vi "Main Interface.vi"() -> ()   [LabVIEW 2015]
uses:
  Ctrls/Data operation control.ctl
  <vilib>/Utility/error.llb/DialogType.ctl
  <vilib>/DAQmx/read.llb/DAQmx Read (Counter U32 1Chan 1Samp).vi
  <vilib>/DAQmx/create/channels.llb/DAQmx Create Channel (CI-Count Edges).vi
  <vilib>/DAQmx/miscellaneous.llb/DAQmx Fill In Error Info.vi
  <vilib>/Waveform/WDTFileIO.llb/Export Waveform To Spreadsheet File.vi
  <resource>/objmgr/daqmx.rc
panel:
  in  "Threshold value (mV)":i16=150
  in  "Source":u16(ring)=1 items=["Channel 1", "Channel 2", "Channel 3", "Channel 4", "Math"]
  out "Waveform Data":waveform(dbl)(graph)
  in  "Output File":path
  in  "Create CSV Output File":bool
  in  "VISA Resource Name":refnum<visa-resource-name>="USB0::0x0957::0x1724::MY50340116::INSTR"
  in  "Timeout Value (ms)":u32=2000
  out "# Points":i32
  in  "# Points (Stop/Single required for >1k)":u16(ring)=3 items=["8M (Single required)", "4M", "2M", "1M", "500k", "200k", "100k", "50k", "20k", "10k", "5k", "2k", "1k", "500", "250", "100"]
  out "error out":errorcluster
  in  "Sample frequency (KHz)":dbl=10.0
  in  "Amplitude":u16(ring)=1 items=["Channel 1", "Channel 2", "Channel 3", "Channel 4", "Math"]
  out "Amplitude (mV)":dbl
  in  "Row add 1":bool
  in  "Tab Control":enum32{"Parameter Setup", "Map", "Data"}(tab)
  in  "Timelapse per pixel (ms)":i32=100
  in  "Size of a single pixel (um)":dbl=2.812
  in  "Quantity of Pixels of one step":dbl=6.0
  in  "X direction total length- Width (um)":dbl=1.15
  in  "Y direction total length- Height (um)":dbl=1.66
  in  "counter":tag="Dev3/ctr2"
  in  "CI.CountEdges.Term":tag="/Dev3/PFI0"
  out "SEE Scanning Map":dbl[][](graph)
  out "Number of Rows":i32
  out "Number of Volumns":i32
  out "Length of each step":dbl
  out "Galvo":bool
  in  "Reset":bool
  in  "stop":bool
  out "Total steps":i32
  in  "Current Step":i32
  out "output array":dbl[][](array[numeric])
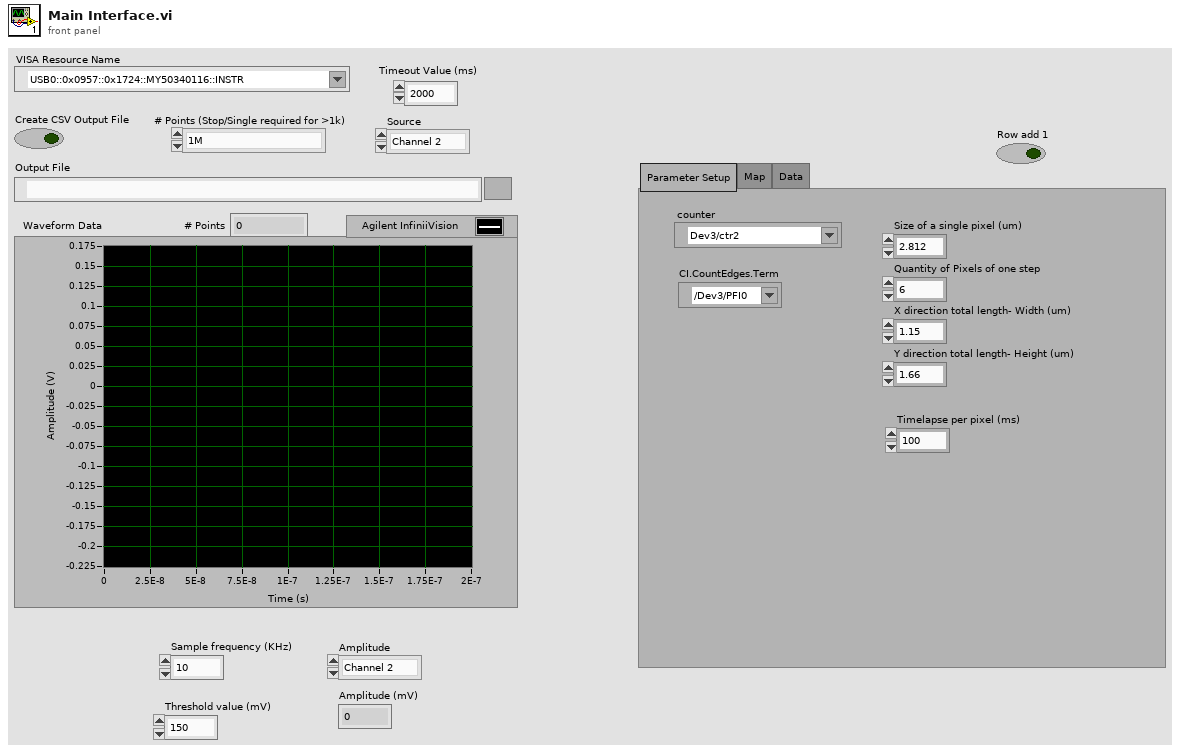
[diagram p1: front panel]
types:
  T1 = typedef "DialogType.ctl" = u16
  T2 = typedef "Data operation control.ctl" = cluster{"States":enum16{"Initializtion", "SEE maping", "Exit"}, "SEE data":i32}
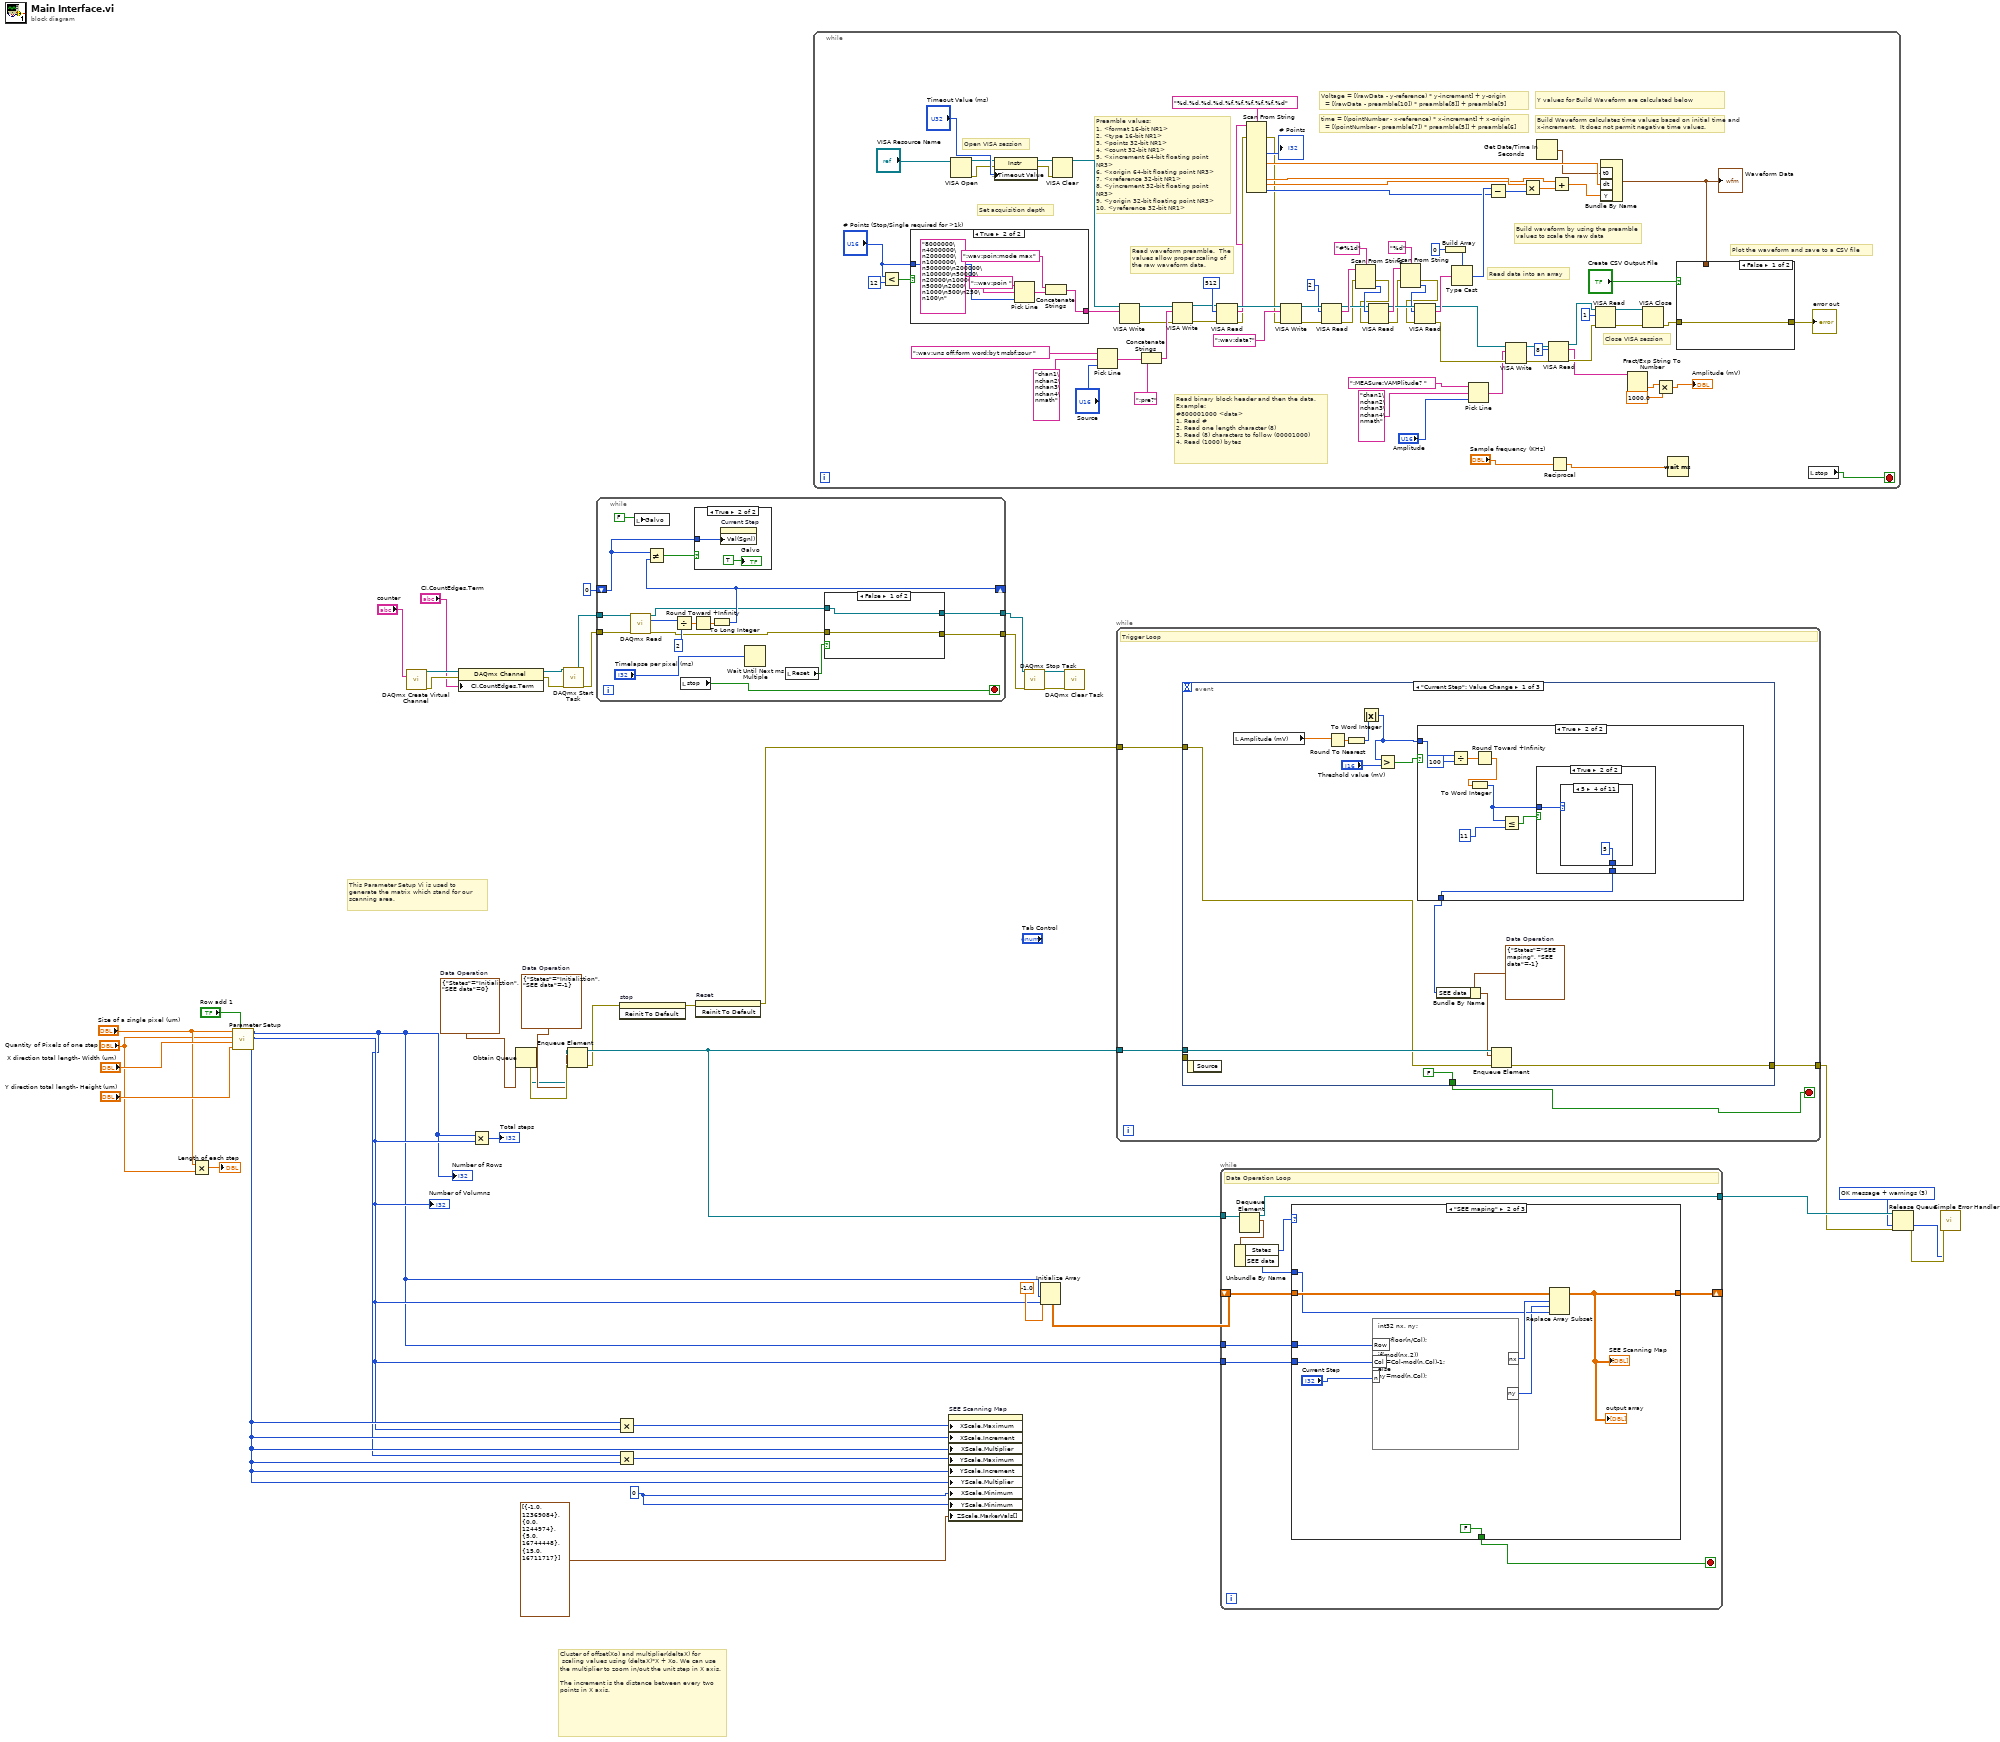
[diagram p0: block diagram]
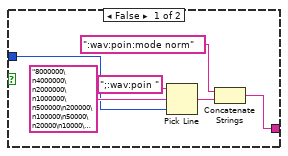
[diagram p2: hidden frame]
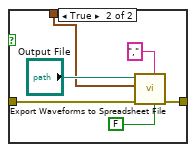
[diagram p3: hidden frame]
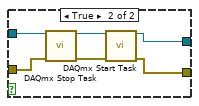
[diagram p4: hidden frame]
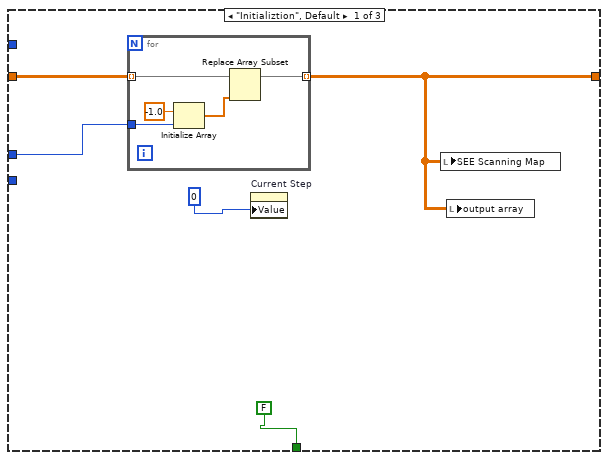
[diagram p6: hidden frame]
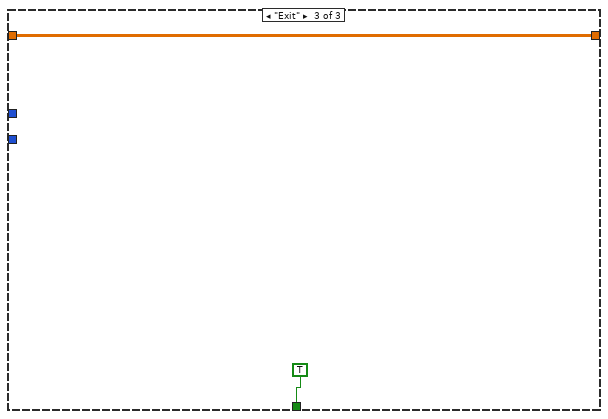
[diagram p7: hidden frame]
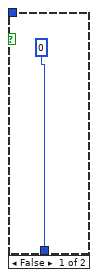
[diagram p8: hidden frame]
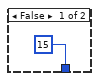
[diagram p9: hidden frame]
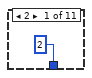
[diagram p10: hidden frame]
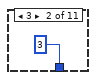
[diagram p11: hidden frame]
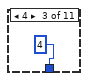
[diagram p12: hidden frame]
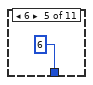
[diagram p13: hidden frame]
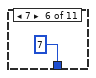
[diagram p14: hidden frame]
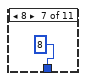
[diagram p15: hidden frame]
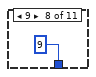
[diagram p16: hidden frame]
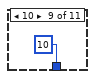
[diagram p17: hidden frame]
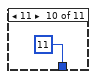
[diagram p18: hidden frame]
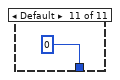
[diagram p19: hidden frame]
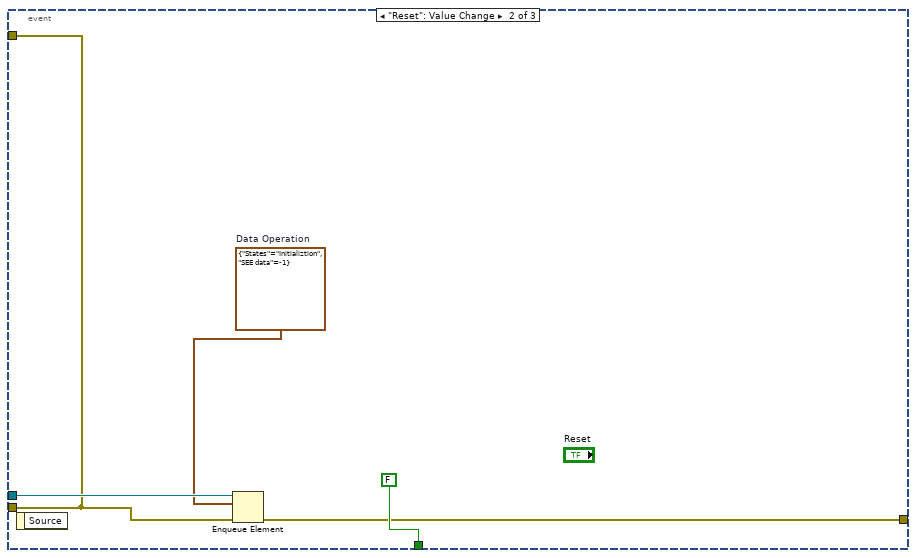
[diagram p20: hidden frame]
diagram:
  w25 = T1 3 items=["no dialog", "OK message", "continue or stop message", "OK message + warnings", "continue/stop + warnings"] ("type of dialog (OK msg:1)")
  w28 = 0
  w37 = T2 {"States"=enum."Initializtion", "SEE data"=-1}  # Data Operation
  w39 = T2 {"States"=enum."Initializtion", "SEE data"=0}  # Data Operation
  # "This Parameter Setup Vi is used to \ngenerate the matrix which stand for our\nscanning area."
  # "Cluster of offset(Xo) and multiplier(deltaX) for\n scaling values using (deltaX)*X + Xo. We can use the multiplier to zoom in/out the unit step in X axis.\n\nThe increment is the distance between every two points in X axis."
  n1 = Multiply(x="Size of a single pixel (um)", y="Quantity of Pixels of one step") -> (x*y=→"Length of each step":dbl)
  n2 = call "Parameter Setup.vi"("Row add 1"="Row add 1", "Y direction total length- Height (um)"="Y direction total length- Height (um)", "X direction total length- Width (um)"="X direction total length- Width (um)", "Quantity of Pixels of one step"="Quantity of Pixels of one step", "Size of a single pixel (um)"="Size of a single pixel (um)") -> ("Length of each Step (um)"=w29:i32, "Number of Volumns"=w3:i32, "Number of Rows"=w2:i32)  [unwired: 4 in]
  "Number of Rows" <- w2
  "Number of Volumns" <- w3
  n3 = call-poly <vilib>:"DAQmx Create Virtual Channel.vi"("counter"="counter") -> ("task out"=w20:refnum<k21>, "error out"=w19:errorcluster)  [unwired: 13 in]
  n4 = property class="DAQmx Channel"(reference=w20, error in=w19, "CI.CountEdges.Term"="CI.CountEdges.Term") -> (reference out=w16:refnum<k21>, error out=w15:errorcluster)
  n5 = Multiply(x=w2, y=w3) -> (x*y=→"Total steps":i32)
  n6 = Obtain Queue(element data type=w39) -> (queue out=w36:refnum<queue>, error out=w38:errorcluster)  [unwired: 4 in, 1 out]
  n7 = call <vilib>:"DAQmx Start Task.vi"("task/channels in"=w16, "error in"=w15) -> ("task out"=w14:refnum<k21>, "error out"=w13:errorcluster)  [unwired: 12 in]
  n8 = Enqueue Element(queue=w36, element=w37, error in (no error)=w38) -> (queue out=w35:refnum<queue>, error out=w7:errorcluster)  [unwired: 1 in, 1 out]
  n9 = while {
    tunnel: w14 -> [w58]
    tunnel: w13 -> [w57]
    shift-right: [w48] -> _
    shift-left: u32 0 ("data") -> [w52]
    tunnel: [w42] -> w11
    tunnel: [w44] -> w9
    stop <- w53 stop-if-true
    n10 = call-poly <vilib>:"DAQmx Read.vi"("task/channels in"=w58, "error in"=w57) -> ("task out"=w46:refnum<k21>, "data"=w56:u32, "error out"=w43:errorcluster)  [unwired: 11 in]
    n11 = local write "Galvo"(FALSE) -> ()
    n12 = Divide(x=w56, y=u32 2) -> (x/y=w50:dbl)
    n13 = local read "stop"() -> (w53:bool)
    n14 = Round Toward +Infinity(x=w50) -> (ceil(x): smallest int >= x=w49:dbl)
    n15 = To Long Integer(number=w49) -> (32bit integer=w48:i32)
    n16 = Not Equal?(x=w52, y=w48) -> (x != y?=w54:bool)
    n17 = case shown="True" w54 {
      tunnel: w52 -> [_ w68]
      frame False {
      }
      frame True {
        n18 = property on="Current Step" class="DigNum (strict)"("Val(Sgnl)"=w68) -> ()  [unwired: 2 in, 2 out]
        "Galvo" <- TRUE
      }
    }
    n19 = Wait Until Next ms Multiple(millisecond multiple="Timelapse per pixel (ms)") -> ()  [unwired: 1 out]
    n20 = local read "Reset"() -> (w45:bool)
    n21 = case shown="False" w45 {
      tunnel: w46 -> [w60 w65]
      tunnel: [w60 w62] -> w44
      tunnel: w43 -> [w59 w66]
      tunnel: [w59 w61] -> w42
      frame False {
      }
      frame True {
        n22 = call <vilib>:"DAQmx Stop Task.vi"("task/channels in"=w65, "error in"=w66) -> ("task out"=w64:refnum<k21>, "error out"=w63:errorcluster)  [unwired: 12 in]
        n23 = call <vilib>:"DAQmx Start Task.vi"("task/channels in"=w64, "error in"=w63) -> ("task out"=w62:refnum<k21>, "error out"=w61:errorcluster)  [unwired: 12 in]
      }
    }
  }
  n24 = Multiply(x=w29, y=w3) -> (x*y=w31:i32)
  n25 = Multiply(x=w2, y=w29) -> (x*y=w30:i32)
  n26 = invoke on="stop" class="Bool (strict)" method="Reinit To Default"(error in=w7) -> (error out=w6:errorcluster)  [unwired: 2 in, 2 out]
  n27 = invoke on="Reset" class="Bool (strict)" method="Reinit To Default"(error in=w6) -> (error out=w5:errorcluster)  [unwired: 2 in, 2 out]
  n28 = while {
    stop <- w69 stop-if-true
    # "Close VISA session"
    # "Open VISA session"
    # "Set acquisition depth"
    # "Plot the waveform and save to a CSV file"
    # "Build Waveform calculates time values based on initial time and x-increment.  It does not permit negative time values."
    # "Y values for Build Waveform are calculated below"
    # "Build waveform by using the preamble values to scale the raw data"
    # "Read data into an array"
    # "Read binary block header and then the data.  Example: \n#800001000 <data>\n1. Read #\n2. Read one length character (8)\n3. Read (8) characters to follow (00001000)\n4. Read (1000) bytes"
    # "Read waveform preamble.  The values allow proper scaling of the raw waveform data."
    # "time = [(pointNumber - x-reference) * x-increment] + x-origin\n\t = [(pointNumber - preamble[7]) * preamble[5]] + preamble[6]"
    # "Voltage = [(rawData - y-reference) * y-increment] + y-origin\n\t\t= [(rawData - preamble[10]) * preamble[8]] + preamble[9]"
    # "Preamble values: \n1. <format 16-bit NR1>\n2. <type 16-bit NR1>\n3. <points 32-bit NR1>\n4. <count 32-bit NR1>\n5. <xincrement 64-bit floating point NR3>\n6. <xorigin 64-bit floating point NR3>\n7. <xreference 32-bit NR1>\n8. <yincrement 32-bit floating point NR3>\n9. <yorigin 32-bit floating point NR3>\n10. <yreference 32-bit NR1>"
    n29 = Less?(x="# Points (Stop/Single required for >1k)", y=u16 12) -> (x < y?=w95:bool)
    n30 = case shown="True" w95 {
      tunnel: [w152 w156] -> w100
      tunnel: "# Points (Stop/Single required for >1k)" -> [w153 w157]
      frame False {
        n31 = Pick Line(string ("")=";:wav:poin ", multi-line string="8000000\n4000000\n2000000\n1000000\n500000\n200000\n100000\n50000\n20000\n10000\n5000\n2000\n1000\n500\n250\n100\n", line index=w153) -> (output string=w151:string)
        n32 = Concatenate Strings(":wav:poin:mode norm" ("string"), w151) -> (w152:string)
      }
      frame True {
        n33 = Pick Line(string ("")=";:wav:poin ", multi-line string="8000000\n4000000\n2000000\n1000000\n500000\n200000\n100000\n50000\n20000\n10000\n5000\n2000\n1000\n500\n250\n100\n", line index=w157) -> (output string=w160:string)
        n34 = Concatenate Strings(":wav:poin:mode max" ("string"), w160) -> (w156:string)
      }
    }
    n35 = VISA Open(VISA resource name="VISA Resource Name") -> (VISA resource name=w105:refnum<visa-resource-name>, error out=w104:errorcluster)  [unwired: 4 in]
    n36 = property class="Instr"(reference=w105, error in=w104, "General Settings:Timeout Value"="Timeout Value (ms)") -> (reference out=w103:refnum<visa-resource-name>, error out=w102:errorcluster)
    n37 = VISA Clear(VISA resource name=w103, error in (no error)=w102) -> (VISA resource name out=w99:refnum<visa-resource-name>)  [unwired: 1 out]
    n38 = Pick Line(string ("")=":wav:uns off;form word;byt msbf;sour ", multi-line string="chan1\nchan2\nchan3\nchan4\nmath", line index="Source") -> (output string=w145:string)
    n39 = VISA Write(VISA resource name=w99, write buffer=w100) -> (VISA resource name out=w98:refnum<visa-resource-name>, error out=w97:errorcluster)  [unwired: 1 in, 1 out]
    n40 = Concatenate Strings(w145, ";pre?" ("string")) -> (w146:string)
    n41 = VISA Write(VISA resource name=w98, write buffer=w146, error in (no error)=w97) -> (VISA resource name out=w142:refnum<visa-resource-name>, error out=w141:errorcluster)  [unwired: 1 out]
    n42 = VISA Read(VISA resource name=w142, byte count=u32 512, error in (no error)=w141) -> (VISA resource name out=w140:refnum<visa-resource-name>, read buffer=w117:string, error out=w93:errorcluster)  [unwired: 1 out]
    n43 = Scan From String(format string="%d,%d,%d,%d,%f,%f,%f,%f,%f,%d", input string=w117, error in=w93) -> (error out=w92:errorcluster, output 3=→"# Points":i32, output 5=w110:dbl, output 8=w122:dbl, output 9=w120:dbl, output 10=w115:i32)  [unwired: 16 in, 2 out]
    n44 = VISA Write(VISA resource name=w140, write buffer=":wav:data?", error in (no error)=w92) -> (VISA resource name out=w138:refnum<visa-resource-name>, error out=w137:errorcluster)  [unwired: 1 out]
    n45 = VISA Read(VISA resource name=w138, byte count=u32 2, error in (no error)=w137) -> (VISA resource name out=w132:refnum<visa-resource-name>, read buffer=w135:string, error out=w91:errorcluster)  [unwired: 1 out]
    n46 = Scan From String(format string="#%1d", input string=w135, error in=w91) -> (error out=w90:errorcluster, output 1=w133:i32)  [unwired: 2 in, 2 out]
    n47 = VISA Read(VISA resource name=w132, byte count=w133, error in (no error)=w90) -> (VISA resource name out=w129:refnum<visa-resource-name>, read buffer=w131:string, error out=w89:errorcluster)  [unwired: 1 out]
    n48 = Scan From String(format string="%d", input string=w131, error in=w89) -> (error out=w88:errorcluster, output 1=w128:i32)  [unwired: 2 in, 2 out]
    n49 = VISA Read(VISA resource name=w129, byte count=w128, error in (no error)=w88) -> (VISA resource name out=w84:refnum<visa-resource-name>, read buffer=w125:string, error out=w81:errorcluster)  [unwired: 1 out]
    n50 = Build Array(i16 0 ("element")) -> (w126:i16[])
    n51 = Type Cast(type=w126, x=w125) -> (*(type *) &x=w116:i16[])
    n52 = Pick Line(string ("")=":MEASure:VAMPlitude? " ("write buffer"), multi-line string="chan1\nchan2\nchan3\nchan4\nmath", line index="Amplitude") -> (output string=w78:string)
    n53 = Subtract(x=w116, y=w115) -> (x-y=w123:i32[])
    n54 = VISA Write(VISA resource name=w84, write buffer=w78, error in (no error)=w81) -> (VISA resource name out=w83:refnum<visa-resource-name>, error out=w80:errorcluster)  [unwired: 1 out]
    n55 = Multiply(x=w122, y=w123) -> (x*y=w121:dbl[])
    n56 = Get Date/Time In Seconds() -> (seconds since 1Jan1904=w109:timestamp)
    n57 = VISA Read(VISA resource name=w83, byte count=u32 8, error in (no error)=w80) -> (VISA resource name out=w82:refnum<visa-resource-name>, read buffer=w73:string, error out=w79:errorcluster)  [unwired: 1 out]
    n58 = Reciprocal(x="Sample frequency (KHz)") -> (1/x=w85:dbl)
    n59 = Add(x=w120, y=w121) -> (x+y=w114:dbl[])
    n60 = VISA Read(VISA resource name=w82, byte count=u32 1, error in (no error)=w79) -> (VISA resource name out=w119:refnum<visa-resource-name>, error out=w118:errorcluster)  [unwired: 2 out]
    n61 = Bundle By Name("t0"=w109, "dt"=w110, "Y"=w114) -> (w108:waveform(dbl))  [unwired: 1 in]
    "Waveform Data" <- w108
    n62 = Fract/Exp String To Number(string=w73) -> (number=w72:dbl)  [unwired: 3 in, 1 out]
    n63 = VISA Close(VISA resource name=w119, error in (no error)=w118) -> (error out=w111:errorcluster)
    n64 = Multiply(x=w72, y=1000.0) -> (x*y=→"Amplitude (mV)":dbl)
    n65 = Wait (ms)(milliseconds to wait=w85) -> ()  [unwired: 1 out]
    n66 = case shown="False" "Create CSV Output File" {
      tunnel: w108 -> [_ w166]
      tunnel: w111 -> [w162 w165]
      tunnel: [w162 w163] -> w87
      frame False {
      }
      frame True {
        n67 = call-poly <vilib>:"Export Waveforms to Spreadsheet File.vi"("header? (write header:T)"=FALSE, "delimiter (Tab)"=",", "error in (no error)"=w165, "waveform"=w166, "file path (dialog if empty)"="Output File") -> ("error out"=w163:errorcluster)  [unwired: 5 in, 1 out]
      }
    }
    "error out" <- w87
    n68 = local read "stop"() -> (w69:bool)
  }
  n69 = property on="SEE Scanning Map" class="IntGraph (strict)"("XScale.Maximum"=w31, "XScale.Increment"=w29, "XScale.Multiplier"=w29, "YScale.Maximum"=w30, "YScale.Increment"=w29, "YScale.Multiplier"=w29, "XScale.Minimum"=w28, "YScale.Minimum"=w28, "ZScale.MarkerVals[]"=cluster{dbl, u32}[] [{-1.0, 12369084}, {0.0, 1244974}, {5.0, 16744448}, {15.0, 16711717}] ("Z Scale.Marker Values[]")) -> ()  [unwired: 2 in, 2 out]
  n70 = call <vilib>:"DAQmx Stop Task.vi"("task/channels in"=w9, "error in"=w11) -> ("task out"=w8:refnum<k21>, "error out"=w10:errorcluster)  [unwired: 12 in]
  n71 = Initialize Array(-1.0 ("element"), w2, w3) -> (w32:dbl[][])
  n72 = call <vilib>:"DAQmx Clear Task.vi"("task in"=w8, "error in"=w10) -> ()  [unwired: 13 in, 1 out]
  n73 = while {
    tunnel: w35 -> [w172]
    tunnel: [w171] -> w4
    tunnel: w5 -> [w169]
    stop <- w170 stop-if-true
    # "Trigger Loop"
    n74 = event shown="[0] \"Current Step\": Value Change" {
      selector: _ -> [_ _ _]
      dyn-events: _ -> [_ _ _]
      timeout: _ -> [_ _ _]
      tunnel: [FALSE FALSE TRUE] -> w170
      tunnel: w172 -> [w184 w213 w218]
      tunnel: [w183 w210 w217] -> w171
      tunnel: [_ w209 w214] -> _
      tunnel: w169 -> [w180 w209 w214]
      event "Current Step": Value Change {
        w182 = T2 {"States"=enum."SEE maping", "SEE data"=-1}  # Data Operation
        n75 = event-data() -> ()  [unwired: 1 in, 1 out]
        n76 = local read "Amplitude (mV)"() -> (w175:dbl)
        n77 = Round To Nearest(number=w175) -> (nearest integer value=w179:dbl)
        n78 = To Word Integer(number=w179) -> (16bit integer=w174:i16)
        n79 = Absolute Value(x=w174) -> (abs(x)=w173:i16)
        n80 = Greater?(x=w173, y="Threshold value (mV)") -> (0:w178:bool)
        n81 = case shown="True" w178 {
          tunnel: [0 w190] -> w177
          tunnel: w173 -> [_ w194]
          frame False {
          }
          frame True {
            n82 = Divide(x=w194, y=i16 100) -> (x/y=w192:dbl)
            n83 = Round Toward +Infinity(x=w192) -> (ceil(x): smallest int >= x=w191:dbl)
            n84 = To Word Integer(number=w191) -> (16bit integer=w189:i16)
            n85 = Less Or Equal?(x=w189, y=11) -> (x <= y?=w187:bool)
            n86 = case shown="True" w187 {
              tunnel: w189 -> [_ w197]
              tunnel: [15 w196] -> w190
              frame False {
              }
              frame True {
                n87 = case shown="5" w197 {
                  tunnel: [2 3 4 5 6 7 8 9 10 11 0] -> w196
                  frame 2 {
                  }
                  frame 3 {
                  }
                  frame 4 {
                  }
                  frame 5 {
                  }
                  frame 6 {
                  }
                  frame 7 {
                  }
                  frame 8 {
                  }
                  frame 9 {
                  }
                  frame 10 {
                  }
                  frame 11 {
                  }
                  frame Default {
                  }
                }
              }
            }
          }
        }
        n88 = Bundle By Name(cluster=w182, "SEE data"=w177) -> (w181:T2)
        n89 = Enqueue Element(queue=w184, element=w181, error in (no error)=w180) -> (error out=w183:errorcluster)  [unwired: 1 in, 2 out]
      }
      event "Reset": Value Change {
        w212 = T2 {"States"=enum."Initializtion", "SEE data"=-1}  # Data Operation
        n90 = event-data() -> ()  [unwired: 1 in, 1 out]
        n91 = Enqueue Element(queue=w213, element=w212, error in (no error)=w209) -> (error out=w210:errorcluster)  [unwired: 1 in, 2 out]
      }
      event "stop": Value Change {
        w216 = T2 {"States"=enum."Exit", "SEE data"=-1}  # Data Operation
        n92 = event-data() -> ()  [unwired: 1 in, 1 out]
        n93 = Enqueue Element(queue=w218, element=w216, error in (no error)=w214) -> (error out=w217:errorcluster)  [unwired: 1 in, 2 out]
      }
    }
  }
  n94 = while {
    tunnel: w35 -> [w228]
    tunnel: [w225] -> w34
    shift-right: [w223] -> _
    shift-left: w32 -> [w224]
    tunnel: w2 -> [w221]
    tunnel: w3 -> [w220]
    stop <- w219 stop-if-true
    # "Data Operation Loop"
    n95 = Dequeue Element(queue=w228) -> (queue out=w225:refnum<queue>, element=w227:T2)  [unwired: 2 in, 2 out]
    n96 = Unbundle By Name(w227) -> ("States"=w226:enum16{"Initializtion", "SEE maping", "Exit"}, "SEE data"=w222:i32)
    n97 = case shown="\"SEE maping\"" w226 {
      tunnel: w224 -> [w232 w244 w249]
      tunnel: [w229 w241 w249] -> w223
      tunnel: w222 -> [_ w242 _]
      tunnel: w221 -> [w233 w246 _]
      tunnel: [FALSE FALSE TRUE] -> w219
      tunnel: w220 -> [_ w245 _]
      frame "Initializtion", Default {
        n98 = for {
          tunnel: w233 -> [w237]
          tunnel: w232 -> [w236] mode=indexing
          tunnel: [w235] -> w229 mode=indexing
          n99 = Initialize Array(-1.0 ("element"), w237) -> (w234:dbl[])
          n100 = Replace Array Subset(array=w236, new element=w234) -> (w235:dbl[])  [unwired: 1 in]
        }
        n101 = property on="Current Step" class="DigNum (strict)"("Value"=u32 0 ("Count")) -> ()  [unwired: 2 in, 2 out]
        n102 = local write "SEE Scanning Map"(w229) -> ()
        n103 = local write "output array"(w229) -> ()
      }
      frame "SEE maping" {
        n104 = formula code="int32 nx, ny;\n\nnx=floor(n/Col); \n\nif(mod(nx,2))\nny=Col-mod(n,Col)-1; \nelse\nny=mod(n,Col);"("Row"=w246, "Col"=w245, "n"="Current Step") -> ("nx"=w243:i32, "ny"=w240:i32)
        n105 = Replace Array Subset(array=w244, new element=w242, index (row)=w243, index (col)=w240) -> (w241:dbl[][])
        "SEE Scanning Map" <- w241
        "output array" <- w241
      }
      frame "Exit" {
      }
    }
  }
  n106 = Release Queue(queue=w34, error in (no error)=w4) -> (error out=w26:errorcluster)  [unwired: 1 in, 2 out]
  n107 = call <vilib>:"Simple Error Handler.vi"("type of dialog (OK msg:1)"=w25, "error in (no error)"=w26) -> ()  [unwired: 3 in, 5 out]
